vi "Acquisition du son.vi"() -> ()   [LabVIEW 2017]
uses:
  <vilib>/Analysis/3filter.llb/Filter Passband Type.ctl
  <vilib>/Analysis/3filter.llb/Butterworth Filter (DBL).vi
  <vilib>/Analysis/NI_AALPro.lvlib
  <vilib>/Analysis/NI_AALBase.lvlib
panel:
  out "K":dbl
  in  "°C":dbl
  out "Graphe 2":dbl[](graph)
  out "Spectre 2":dbl[](graph)
  out "Spectre":dbl[](graph)
  in  "fc":dbl
  in  "Ordre filtre":dbl min=0.0 step=1.0
  out "Graphe":dbl[](graph)
  in  "stop":bool
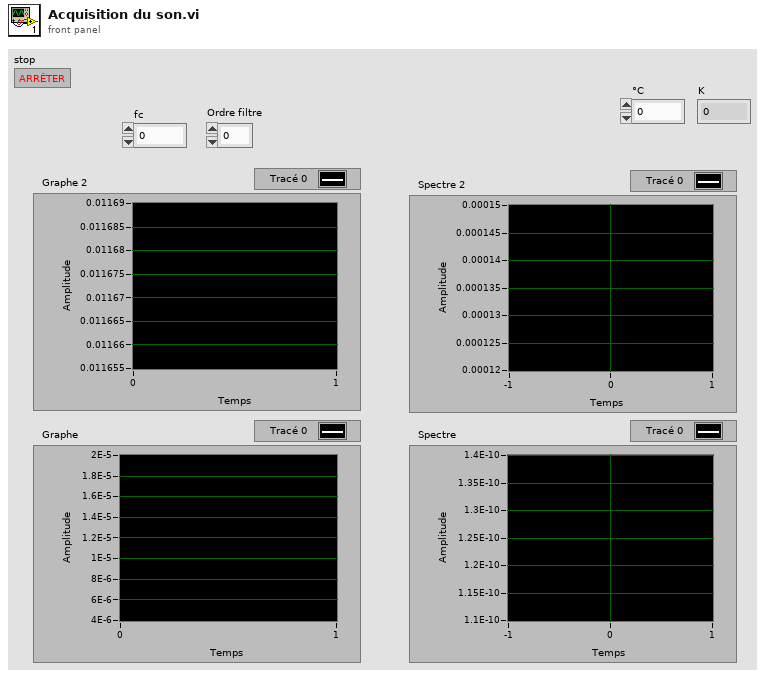
[diagram p1: front panel]
types:
  T1 = typedef "NI_AALBase.lvlib/Filter Passband Type.ctl" = enum32{"Lowpass", "Highpass", "Bandpass", "Bandstop"}
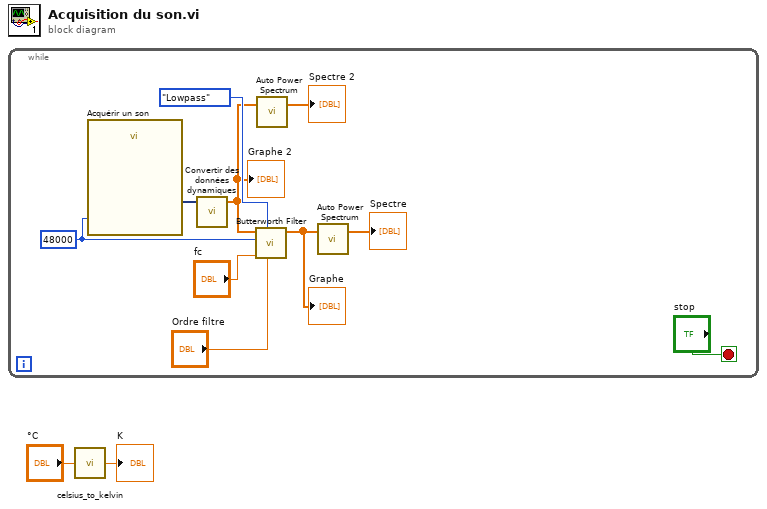
[diagram p0: block diagram]
diagram:
  n1 = while {
    stop <- "stop" stop-if-true
    w4 = 48000
    n2 = call "Acquérir un son"("Sample rate (Hz)"=w4) -> ("Data"=w5:dynamicdata)  [unwired: 17 in, 1 out]
    n3 = call "Convertir des données dynamiques"("Dynamic Data Type"=w5) -> ("Array"=w6:dbl[])  [unwired: 3 in]
    "Graphe 2" <- w6
    n4 = call-poly <vilib>:"Butterworth Filter.vi"("order"="Ordre filtre", "filter type"=Filter_Passband_Type."Lowpass", "low cutoff freq: fl"="fc", "sampling freq: fs"=w4, "X"=w6) -> ("Filtered X"=w3:dbl[])  [unwired: 3 in, 1 out]
    "Graphe" <- w3
    n5 = call <vilib>:"Auto Power Spectrum.vi"("Signal (V)"=w6) -> ("Power Spectrum (V^2 rms)"=→"Spectre 2":dbl[])  [unwired: 1 in, 1 out]
    n6 = call <vilib>:"Auto Power Spectrum.vi"("Signal (V)"=w3) -> ("Power Spectrum (V^2 rms)"=→"Spectre":dbl[])  [unwired: 1 in, 1 out]
  }
  n7 = call "celsius_to_kelvin.vi"("°C"="°C") -> ("K"=→"K":dbl)
